vi "gaussmeter read values.vi"(8 "error in (no error)":errorcluster, 11 "VISA resource name":refnum<visa-resource-name>="GPIB1::11::INSTR") -> (0 "error out":errorcluster, 2 "gaussmeter reading":T1, 3 "VISA resource name":refnum<visa-resource-name>)   [LabVIEW 2013]
uses:
  magnet/magnet cartesian field.ctl
panel:
  out "debug string 4":string
  out "debug string 3":string
  out "debug string 2":string
  out "debug string":string
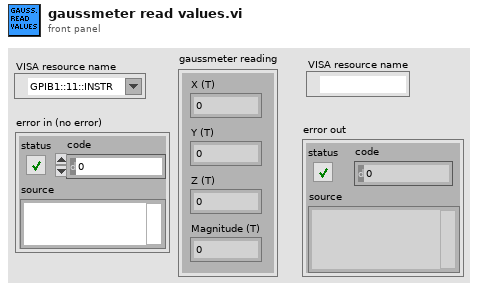
[diagram p1: front panel]
types:
  T1 = typedef "magnet cartesian field.ctl" = cluster{"X (T)":dbl, "Y (T)":dbl, "Z (T)":dbl, "Magnitude (T)":dbl}
  T2 = cluster{"X (T)":dbl, "Y (T)":dbl, "Z (T)":dbl, "Vector (T)":dbl}
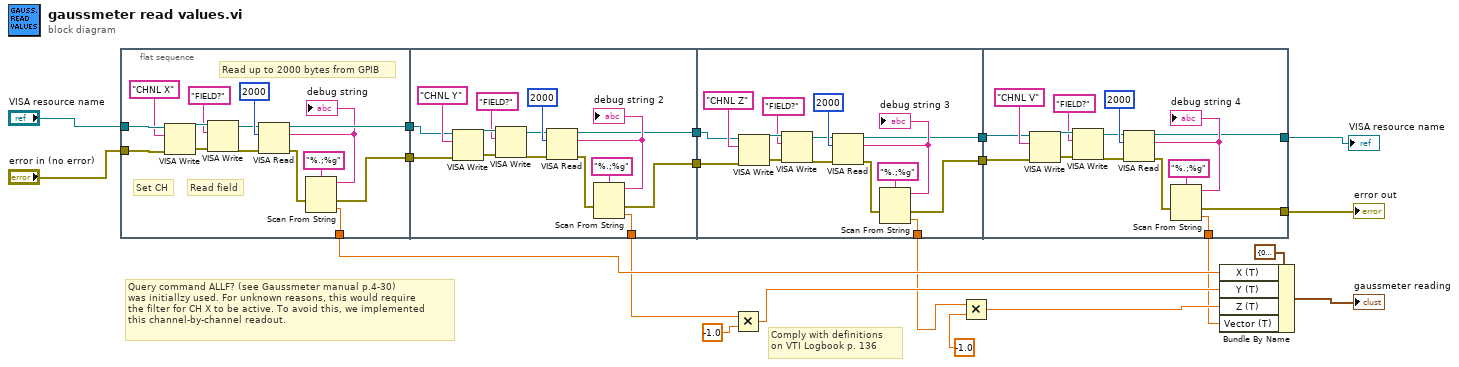
[diagram p0: block diagram]
diagram:
  # "Query command ALLF? (see Gaussmeter manual p.4-30)\nwas initiallzy used. For unknown reasons, this would require \nthe filter for CH X to be active. To avoid this, we implemented\nthis channel-by-channel readout."
  # "Comply with definitions \non VTI Logbook p. 136"
  n1 = flat-sequence {
    tunnel: "VISA resource name" -> [w35]
    tunnel: "error in (no error)" -> [w34]
    tunnel: [w28] -> w17
    tunnel: [w31] -> w12
    tunnel: [w26] -> w11
    tunnel: w12 -> [w40]
    tunnel: w11 -> [w39]
    tunnel: [w38] -> w10
    tunnel: [w37] -> w9
    tunnel: [w36] -> w8
    tunnel: w10 -> [w55]
    tunnel: w9 -> [w54]
    tunnel: [w53] -> w6
    tunnel: [w52] -> w3
    tunnel: [w51] -> w2
    tunnel: [w67] -> w4
    tunnel: [w68] -> w5
    tunnel: w3 -> [w69]
    tunnel: w2 -> [w70]
    tunnel: [w66] -> w1
    frame #0 {
      # "Read field"
      # "Set CH"
      # "Read up to 2000 bytes from GPIB"
      n2 = VISA Write(VISA resource name=w35, write buffer="CHNL X", error in (no error)=w34) -> (VISA resource name out=w22:refnum<visa-resource-name>, error out=w23:errorcluster)  [unwired: 1 out]
      n3 = VISA Write(VISA resource name=w22, write buffer="FIELD?", error in (no error)=w23) -> (VISA resource name out=w25:refnum<visa-resource-name>, error out=w24:errorcluster)  [unwired: 1 out]
      n4 = VISA Read(VISA resource name=w25, byte count=2000, error in (no error)=w24) -> (VISA resource name out=w31:refnum<visa-resource-name>, read buffer=w30:string, error out=w27:errorcluster)  [unwired: 1 out]
      "debug string" <- w30
      n5 = Scan From String(format string="%.;%g", input string=w30, error in=w27) -> (error out=w26:errorcluster, output 1=w28:dbl)  [unwired: 2 in, 2 out]
    }
    frame #1 {
      n6 = VISA Write(VISA resource name=w40, write buffer="CHNL Y", error in (no error)=w39) -> (VISA resource name out=w42:refnum<visa-resource-name>, error out=w43:errorcluster)  [unwired: 1 out]
      n7 = VISA Write(VISA resource name=w42, write buffer="FIELD?", error in (no error)=w43) -> (VISA resource name out=w45:refnum<visa-resource-name>, error out=w44:errorcluster)  [unwired: 1 out]
      n8 = VISA Read(VISA resource name=w45, byte count=2000, error in (no error)=w44) -> (VISA resource name out=w38:refnum<visa-resource-name>, read buffer=w48:string, error out=w46:errorcluster)  [unwired: 1 out]
      "debug string 2" <- w48
      n9 = Scan From String(format string="%.;%g", input string=w48, error in=w46) -> (error out=w37:errorcluster, output 1=w36:dbl)  [unwired: 2 in, 2 out]
    }
    frame #2 {
      n10 = VISA Write(VISA resource name=w55, write buffer="CHNL Z", error in (no error)=w54) -> (VISA resource name out=w57:refnum<visa-resource-name>, error out=w58:errorcluster)  [unwired: 1 out]
      n11 = VISA Write(VISA resource name=w57, write buffer="FIELD?", error in (no error)=w58) -> (VISA resource name out=w60:refnum<visa-resource-name>, error out=w59:errorcluster)  [unwired: 1 out]
      n12 = VISA Read(VISA resource name=w60, byte count=2000, error in (no error)=w59) -> (VISA resource name out=w52:refnum<visa-resource-name>, read buffer=w63:string, error out=w61:errorcluster)  [unwired: 1 out]
      "debug string 3" <- w63
      n13 = Scan From String(format string="%.;%g", input string=w63, error in=w61) -> (error out=w51:errorcluster, output 1=w53:dbl)  [unwired: 2 in, 2 out]
    }
    frame #3 {
      n14 = VISA Write(VISA resource name=w69, write buffer="CHNL V", error in (no error)=w70) -> (VISA resource name out=w72:refnum<visa-resource-name>, error out=w73:errorcluster)  [unwired: 1 out]
      n15 = VISA Write(VISA resource name=w72, write buffer="FIELD?", error in (no error)=w73) -> (VISA resource name out=w75:refnum<visa-resource-name>, error out=w74:errorcluster)  [unwired: 1 out]
      n16 = VISA Read(VISA resource name=w75, byte count=2000, error in (no error)=w74) -> (VISA resource name out=w68:refnum<visa-resource-name>, read buffer=w78:string, error out=w76:errorcluster)  [unwired: 1 out]
      "debug string 4" <- w78
      n17 = Scan From String(format string="%.;%g", input string=w78, error in=w76) -> (error out=w67:errorcluster, output 1=w66:dbl)  [unwired: 2 in, 2 out]
    }
  }
  n18 = Multiply(x=w8, y=-1.0) -> (x*y=w14:dbl)
  n19 = Multiply(x=w6, y=-1.0) -> (x*y=w7:dbl)
  n20 = Bundle By Name(cluster=T2 {"X (T)"=0.0, "Y (T)"=0.0, "Z (T)"=0.0, "Vector (T)"=0.0} ("gaussmeter reading"), "X (T)"=w17, "Y (T)"=w14, "Z (T)"=w7, "Vector (T)"=w1) -> (→"gaussmeter reading":T2)
  "VISA resource name" <- w5
  "error out" <- w4
